vi "题目四.vi"() -> ()   [LabVIEW 2017]
uses:
  <vilib>/measure/NI_MABase.lvlib
panel:
  out "最小值":dbl
  out "dt":dbl
  out "Y":dbl[](array[numeric])
  in  "sampling info":cluster{"Fs":dbl, "#s":dbl}={"Fs"=1000.0, "#s"=1000.0} caption="采样信息" {"Fs" format="%.2p"}
  in  "frequency":dbl=10.0 caption="频率" format="%.2p"
  in  "amplitude":dbl=1.0 caption="幅值" format="%.2p"
  in  "phase":dbl caption="相位" format="%.2p"
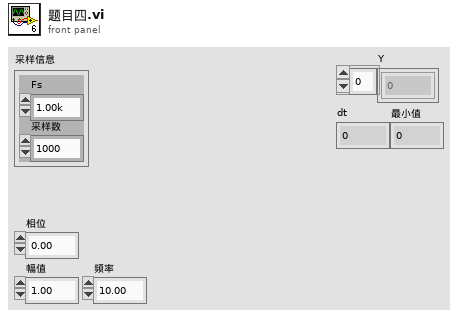
[diagram p1: front panel]
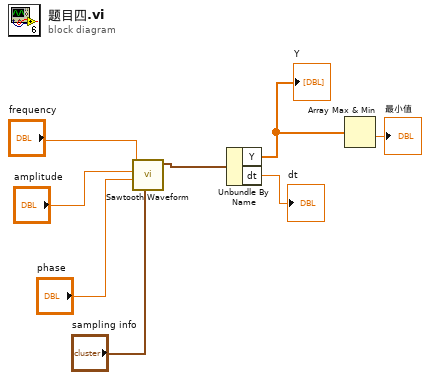
[diagram p0: block diagram]
diagram:
  n1 = call <vilib>:"Sawtooth Waveform.vi"("sampling info"="sampling info", "phase"="phase", "amplitude"="amplitude", "frequency"="frequency") -> ("signal out"=w5:waveform(dbl))  [unwired: 6 in, 1 out]
  n2 = Unbundle By Name(w5) -> ("Y"=w1:dbl[], "dt"=→"dt":dbl)
  "Y" <- w1
  n3 = Array Max & Min(array=w1) -> (min value=→"最小值":dbl)  [unwired: 3 out]
